vi "Response Timeout.vi"(5 "error source class name":string, 7 "error source vi name":string, 8 "error in (no error)":errorcluster, 11 "Interface in":refnum<class "Interface.lvclass">) -> (0 "error out":errorcluster, 3 "Interface out":refnum<class "Interface.lvclass">)   [LabVIEW 2017, in "DSF Core.lvlib" / "Interface.lvclass"]
uses:
  Interface/Interface.lvclass
  Interface/Errors.ctl
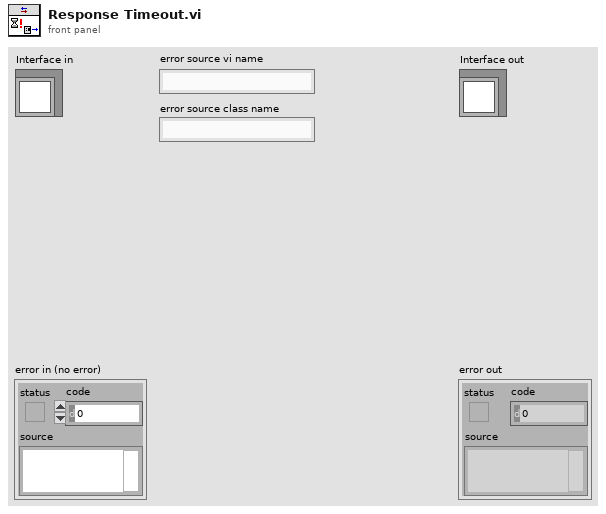
[diagram p1: front panel]
types:
  T1 = typedef "DSF Core.lvlib/Interface.lvclass/Errors.ctl" = enum16{"Command Timeout", "Response Timeout", "Error Timeout", "Invalid Response", "Invalid Response Parameters"}
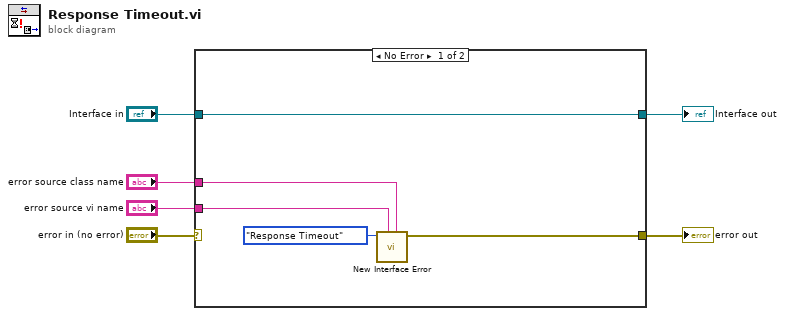
[diagram p0: block diagram]
diagram:
  n1 = case shown="No Error" "error in (no error)" {
    selector: "error in (no error)" -> [_ w12]
    tunnel: "Interface in" -> [w8 w13]
    tunnel: [w8 w13] -> w4
    tunnel: [w11 w12] -> w3
    tunnel: "error source vi name" -> [w10 _]
    tunnel: "error source class name" -> [w7 _]
    frame No Error {
      n2 = call "New Interface Error.vi"("error source class name"=w7, "error source vi name"=w10, "error"=Errors."Response Timeout") -> ("error out"=w11:errorcluster)  [unwired: 7 in, 1 out]
    }
    frame Error {
    }
  }
  "error out" <- w3
  "Interface out" <- w4
